vi "popUPInsertarTuplaEnDBImagen.vi"() -> (2 "datosProducto":cluster{"od":string, "sg":string, "lt":string}, 3 "Listo Ingresar OD SteelGrade Lote":bool=TRUE)   [LabVIEW 2014]
panel:
  in  "textoFinCarga":string="Gracias por ingresar los datos del producto"
  in  "ingresarLote":string="numLote"
  in  "ingresarSteelGrade":string="numSteelGrade"
  in  "ingresarOD":string="numeroOD"
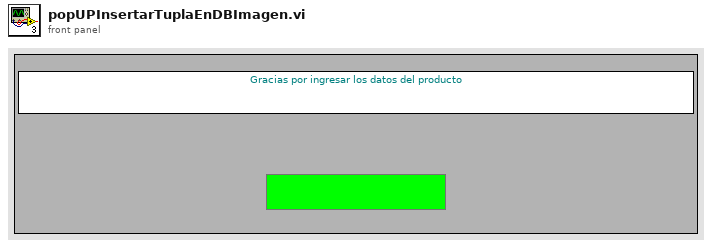
[diagram p1: front panel]
types:
  T1 = enum8{"Enabled", "Disabled", "Disabled and Grayed Out"}
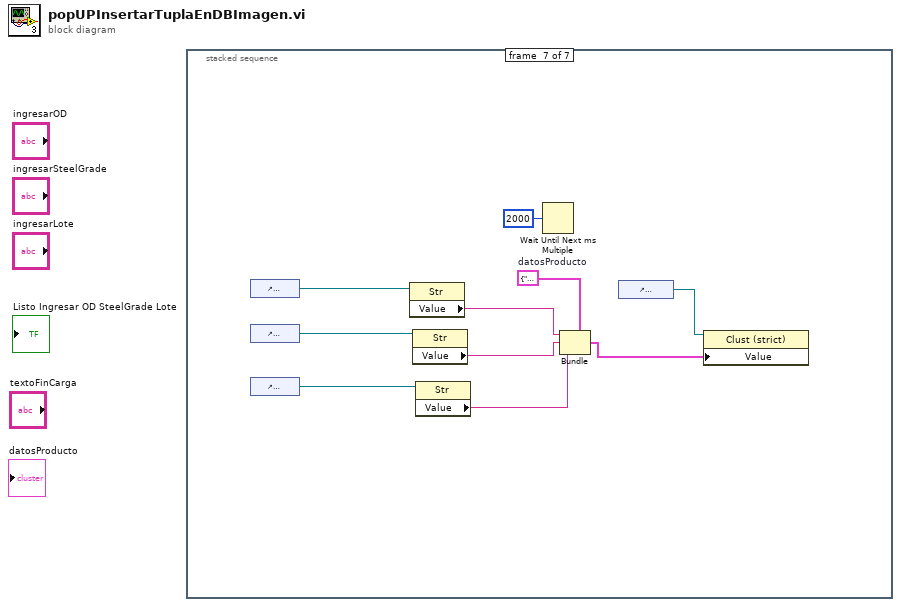
[diagram p0: block diagram]
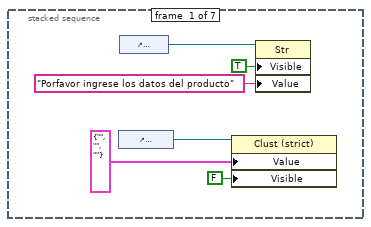
[diagram p2: hidden frame]
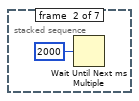
[diagram p3: hidden frame]
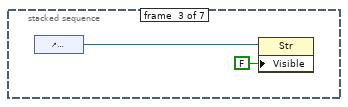
[diagram p4: hidden frame]
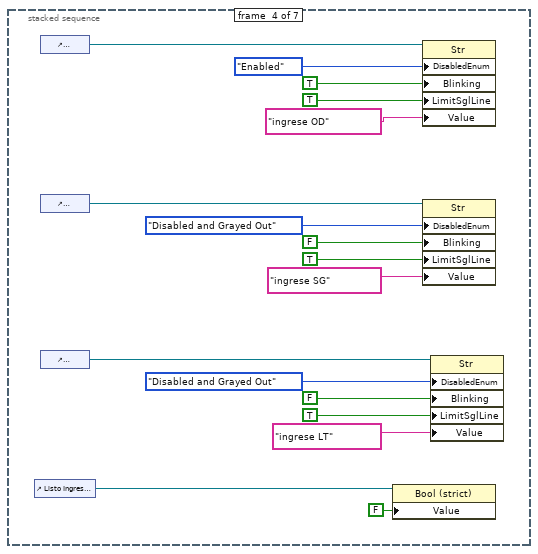
[diagram p5: hidden frame]
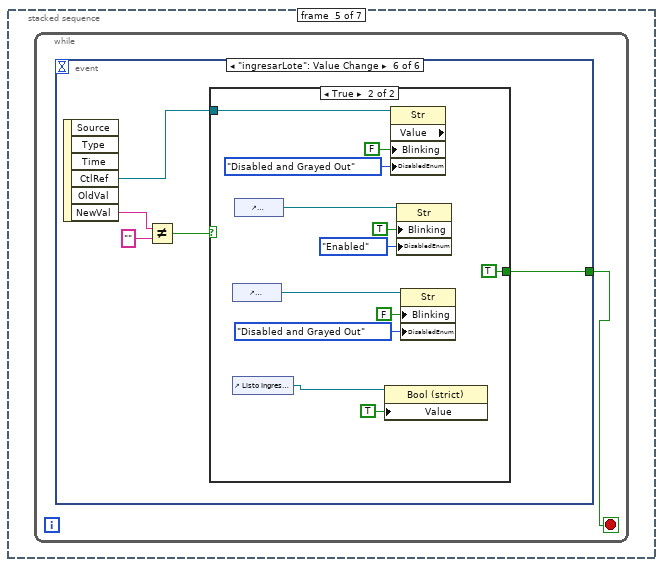
[diagram p6: hidden frame]
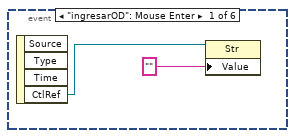
[diagram p7: hidden frame]
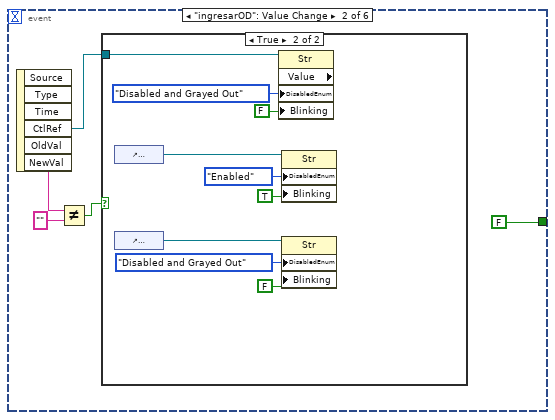
[diagram p8: hidden frame]
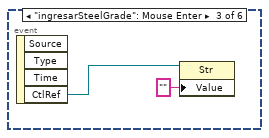
[diagram p10: hidden frame]
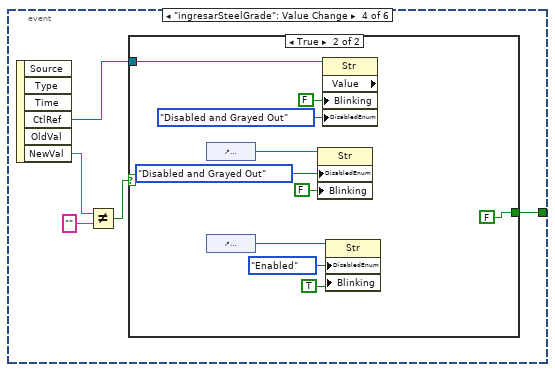
[diagram p11: hidden frame]
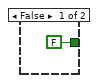
[diagram p12: hidden frame]
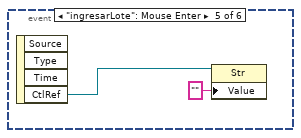
[diagram p13: hidden frame]
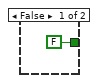
[diagram p14: hidden frame]
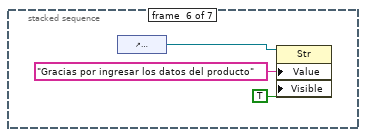
[diagram p15: hidden frame]
diagram:
  n1 = stacked-sequence {
    frame #0 {
      n2 = control-ref of="datosProducto"() -> (w3:refnum<vi>)
      n3 = control-ref of="textoFinCarga"() -> (w6:refnum<vi>)
      n4 = property class="Clust (strict)"(reference=w3, "Value"=cluster{"od":string, "sg":string, "lt":string} {"od"="", "sg"="", "lt"=""}, "Visible"=FALSE) -> ()  [unwired: 1 in, 2 out]
      n5 = property class="Str"(reference=w6, "Visible"=TRUE, "Value"="Porfavor ingrese los datos del producto") -> ()  [unwired: 1 in, 2 out]
    }
    frame #1 {
      n6 = Wait Until Next ms Multiple(millisecond multiple=u32 2000) -> ()  [unwired: 1 out]
    }
    frame #2 {
      n7 = control-ref of="textoFinCarga"() -> (w9:refnum<vi>)
      n8 = property class="Str"(reference=w9, "Visible"=FALSE) -> ()  [unwired: 1 in, 2 out]
    }
    frame #3 {
      n9 = control-ref of="Listo Ingresar OD SteelGrade Lote"() -> (w14:refnum<vi>)
      n10 = control-ref of="ingresarOD"() -> (w26:refnum<vi>)
      n11 = control-ref of="ingresarSteelGrade"() -> (w24:refnum<vi>)
      n12 = control-ref of="ingresarLote"() -> (w22:refnum<vi>)
      n13 = property class="Bool (strict)"(reference=w14, "Value"=FALSE) -> ()  [unwired: 1 in, 2 out]
      n14 = property class="Str"(reference=w26, "DisabledEnum"=T1."Enabled" ("Disabled"), "Blinking"=TRUE, "LimitSglLine"=TRUE ("Limit To Single Line?"), "Value"="ingrese OD") -> ()  [unwired: 1 in, 2 out]
      n15 = property class="Str"(reference=w24, "DisabledEnum"=T1."Disabled and Grayed Out" ("Disabled"), "Blinking"=FALSE, "LimitSglLine"=TRUE ("Limit To Single Line?"), "Value"="ingrese SG") -> ()  [unwired: 1 in, 2 out]
      n16 = property class="Str"(reference=w22, "DisabledEnum"=T1."Disabled and Grayed Out" ("Disabled"), "Blinking"=FALSE, "LimitSglLine"=TRUE ("Limit To Single Line?"), "Value"="ingrese LT") -> ()  [unwired: 1 in, 2 out]
    }
    frame #4 {
      n17 = while {
        stop <- w27 stop-if-true
        n18 = event shown="[5] \"ingresarLote\": Value Change" {
          selector: _ -> [_ _ _ _ _ _]
          dyn-events: _ -> [_ _ _ _ _ _]
          timeout: _ -> [_ _ _ _ _ _]
          tunnel: [_ FALSE _ w49 _ w67] -> w27
          event "ingresarOD": Mouse Enter {
            n19 = event-data() -> ("CtlRef"=w29:refnum<vi>)  [unwired: 1 in, 3 out]
            n20 = property class="Str"(reference=w29, "Value"="") -> ()  [unwired: 1 in, 2 out]
          }
          event "ingresarOD": Value Change {
            n21 = event-data() -> ("CtlRef"=w34:refnum<vi>, "NewVal"=w31:string)  [unwired: 1 in, 4 out]
            n22 = Not Equal?(x=w31, y="") -> (x != y?=w32:bool)
            n23 = case shown="True" w32 {
              tunnel: w34 -> [_ w43]
              frame False {
              }
              frame True {
                n24 = control-ref of="ingresarSteelGrade"() -> (w40:refnum<vi>)
                n25 = control-ref of="ingresarLote"() -> (w37:refnum<vi>)
                n26 = property class="Str" props=["Value", "DisabledEnum", "Blinking"](reference=w43, "DisabledEnum"=T1."Disabled and Grayed Out" ("Disabled"), "Blinking"=FALSE) -> ()  [unwired: 1 in, 3 out]
                n27 = property class="Str"(reference=w40, "DisabledEnum"=T1."Enabled" ("Disabled"), "Blinking"=TRUE) -> ()  [unwired: 1 in, 2 out]
                n28 = property class="Str"(reference=w37, "DisabledEnum"=T1."Disabled and Grayed Out" ("Disabled"), "Blinking"=FALSE) -> ()  [unwired: 1 in, 2 out]
              }
            }
          }
          event "ingresarSteelGrade": Mouse Enter {
            n29 = event-data() -> ("CtlRef"=w45:refnum<vi>)  [unwired: 1 in, 3 out]
            n30 = property class="Str"(reference=w45, "Value"="") -> ()  [unwired: 1 in, 2 out]
          }
          event "ingresarSteelGrade": Value Change {
            n31 = event-data() -> ("CtlRef"=w50:refnum<vi>, "NewVal"=w48:string)  [unwired: 1 in, 4 out]
            n32 = Not Equal?(x=w48, y="") -> (x != y?=w46:bool)
            n33 = case shown="True" w46 {
              tunnel: w50 -> [_ w61]
              tunnel: [FALSE FALSE] -> w49
              frame False {
              }
              frame True {
                n34 = control-ref of="ingresarOD"() -> (w59:refnum<vi>)
                n35 = control-ref of="ingresarLote"() -> (w56:refnum<vi>)
                n36 = property class="Str"(reference=w59, "DisabledEnum"=T1."Disabled and Grayed Out" ("Disabled"), "Blinking"=FALSE) -> ()  [unwired: 1 in, 2 out]
                n37 = property class="Str" props=["Value", "Blinking", "DisabledEnum"](reference=w61, "Blinking"=FALSE, "DisabledEnum"=T1."Disabled and Grayed Out" ("Disabled")) -> ()  [unwired: 1 in, 3 out]
                n38 = property class="Str"(reference=w56, "DisabledEnum"=T1."Enabled" ("Disabled"), "Blinking"=TRUE) -> ()  [unwired: 1 in, 2 out]
              }
            }
          }
          event "ingresarLote": Mouse Enter {
            n39 = event-data() -> ("CtlRef"=w63:refnum<vi>)  [unwired: 1 in, 3 out]
            n40 = property class="Str"(reference=w63, "Value"="") -> ()  [unwired: 1 in, 2 out]
          }
          event "ingresarLote": Value Change {
            n41 = event-data() -> ("CtlRef"=w68:refnum<vi>, "NewVal"=w66:string)  [unwired: 1 in, 4 out]
            n42 = Not Equal?(x=w66, y="") -> (x != y?=w65:bool)
            n43 = case shown="True" w65 {
              tunnel: w68 -> [_ w81]
              tunnel: [FALSE TRUE] -> w67
              frame False {
              }
              frame True {
                n44 = control-ref of="ingresarSteelGrade"() -> (w74:refnum<vi>)
                n45 = control-ref of="Listo Ingresar OD SteelGrade Lote"() -> (w71:refnum<vi>)
                n46 = control-ref of="ingresarOD"() -> (w77:refnum<vi>)
                n47 = property class="Bool (strict)"(reference=w71, "Value"=TRUE) -> ()  [unwired: 1 in, 2 out]
                n48 = property class="Str" props=["Value", "Blinking", "DisabledEnum"](reference=w81, "Blinking"=FALSE, "DisabledEnum"=T1."Disabled and Grayed Out" ("Disabled")) -> ()  [unwired: 1 in, 3 out]
                n49 = property class="Str"(reference=w77, "Blinking"=TRUE, "DisabledEnum"=T1."Enabled" ("Disabled")) -> ()  [unwired: 1 in, 2 out]
                n50 = property class="Str"(reference=w74, "Blinking"=FALSE, "DisabledEnum"=T1."Disabled and Grayed Out" ("Disabled")) -> ()  [unwired: 1 in, 2 out]
              }
            }
          }
        }
      }
    }
    frame #5 {
      n51 = control-ref of="textoFinCarga"() -> (w84:refnum<vi>)
      n52 = property class="Str"(reference=w84, "Value"="Gracias por ingresar los datos del producto", "Visible"=TRUE) -> ()  [unwired: 1 in, 2 out]
    }
    frame #6 {
      w87 = cluster{"od":string, "sg":string, "lt":string} {"od"="", "sg"="", "lt"=""}  # datosProducto
      n53 = control-ref of="ingresarOD"() -> (w93:refnum<vi>)
      n54 = control-ref of="ingresarSteelGrade"() -> (w92:refnum<vi>)
      n55 = control-ref of="ingresarLote"() -> (w91:refnum<vi>)
      n56 = property class="Str"(reference=w93) -> ("Value"=w90:string)  [unwired: 1 in, 2 out]
      n57 = property class="Str"(reference=w92) -> ("Value"=w89:string)  [unwired: 1 in, 2 out]
      n58 = property class="Str"(reference=w91) -> ("Value"=w88:string)  [unwired: 1 in, 2 out]
      n59 = Wait Until Next ms Multiple(millisecond multiple=u32 2000) -> ()  [unwired: 1 out]
      n60 = Bundle(cluster=w87, "od"=w90, "sg"=w89, "lt"=w88) -> (w85:cluster{"od":string, "sg":string, "lt":string})
      n61 = control-ref of="datosProducto"() -> (w86:refnum<vi>)
      n62 = property class="Clust (strict)"(reference=w86, "Value"=w85) -> ()  [unwired: 1 in, 2 out]
    }
  }
